vi "PID Sine Wave.vi"() -> ()   [LabVIEW 2017]
uses:
  <vilib>/addons/control/pid/pid.llb/PID (DBL).vi
  <vilib>/addons/control/pid/NI_PID_pid.lvlib
panel:
  in  "PID gains":T1={"proportional gain (Kc)"=1.0, "integral time (Ti, min)"=0.01, "derivative time (Td, min)"=0.0} {"derivative time (Td, min)" format="%.3f"; "integral time (Ti, min)" format="%.3f"; "proportional gain (Kc)" format="%.3f"}
  in  "Stop VI":bool
  out "Counter Value":T2(graph)
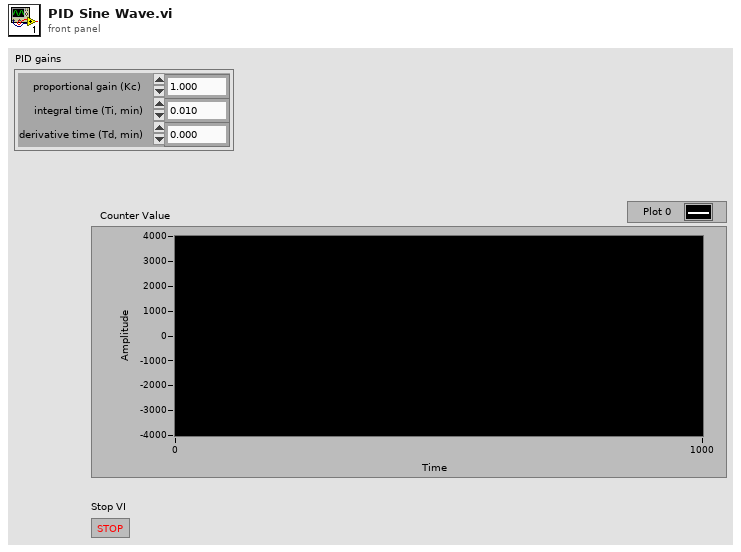
[diagram p1: front panel]
types:
  T1 = cluster{"proportional gain (Kc)":dbl, "integral time (Ti, min)":dbl, "derivative time (Td, min)":dbl}
  T2 = cluster{"Counter Value":dbl, "Counter Value":dbl}
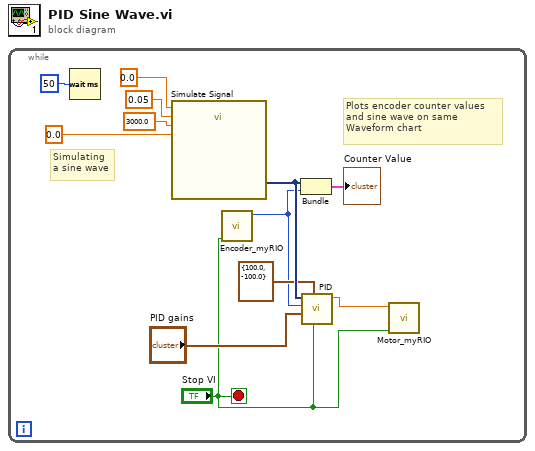
[diagram p0: block diagram]
diagram:
  n1 = while {
    stop <- "Stop VI" stop-if-true
    # "Plots encoder counter values \nand sine wave on same \nWaveform chart"
    # "Simulating\na sine wave"
    n2 = Wait (ms)(milliseconds to wait=u32 50) -> ()  [unwired: 1 out]
    n3 = call "Simulate Signal"("Offset"=0.0, "Frequency"=0.05, "Amplitude"=3000.0, "Phase"=0.0) -> ("Sine"=w6:dynamicdata)  [unwired: 10 in, 1 out]
    n4 = call "Encoder_myRIO.vi"("Reset"="Stop VI") -> ("Counter Value"=w2:i32)  [unwired: 8 in, 1 out]
    n5 = Bundle("Sine"=w6, "Counter Value"=w2) -> (→"Counter Value":cluster{"Sine":dynamicdata, "Counter Value":i32})  [unwired: 1 in]
    n6 = call-poly <vilib>:"PID.vi"("reinitialize? (F)"="Stop VI", "output range"=cluster{"output high":dbl, "output low":dbl} {"output high"=100.0, "output low"=-100.0}, "PID gains"="PID gains", "process variable"=w2, "setpoint"=w6) -> ("output"=w4:dbl)  [unwired: 5 in, 1 out]
    n7 = call "Motor_myRIO.vi"("Stop VI"="Stop VI", "Duty Cycle (-100 to +100)"=w4) -> ()  [unwired: 10 in]
  }
